vi "All Node Groups.vi"(8 "error in (no error)":errorcluster, 10 "Node Name":string, 11 "ChannelService in":refnum<class "ChannelService.lvclass">) -> (0 "error out":errorcluster, 2 "Node Groups":refnum<class "Group.lvclass">[](array[class]), 3 "ChannelService out":refnum<class "ChannelService.lvclass">)   [LabVIEW 2020, in "Vecto.lvlib" / "ChannelService.lvclass"]
uses:
  ChannelService.lvclass
  Group/Group.lvclass
  GroupsAbstractValue/GroupsAbstractValue.lvclass
  C:/dev/lv20CE/relink/lv-promises/Promises/Value/Value.lvclass
  Lookup Group Data.ctl
  Lookup Type.ctl
  lv-promises/Promises/Promise/Promise.lvclass
  ChannelService.lvclass/ChannelService.ctl
  lv-promises/Promises/Promise/Promise.lvclass/Promise.ctl
  lv-promises/Promises/Future/Future.lvclass/Future.ctl
  GroupsAbstractValue/GroupsAbstractValue.lvclass/GroupsAbstractValue.ctl
  lv-promises/Promises/Future/Future.lvclass
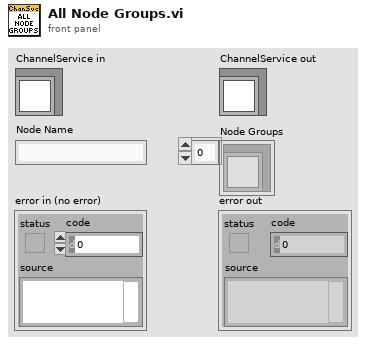
[diagram p1: front panel]
types:
  T1 = typedef "Vecto.lvlib/ChannelService.lvclass/Lookup Type.ctl" = enum16{"Name", "Node", "Pattern"}
  T2 = typedef "Vecto.lvlib/ChannelService.lvclass/Lookup Group Data.ctl" = cluster{"Type":T1, "Group Lookup":string, "Node Lookup":string, "Promise":refnum<class "Promise.lvclass">}
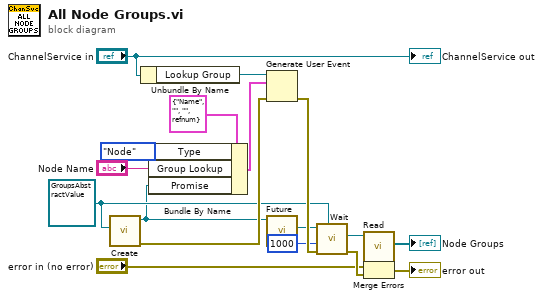
[diagram p0: block diagram]
diagram:
  w11 = refnum<class "GroupsAbstractValue.lvclass"> refnum ("Vecto.lvlib:GroupsValue.lvclass")
  n1 = call "Create.vi"("Result Type"=w11) -> ("error out"=w14:errorcluster, "Promise"=w6:refnum<class "Promise.lvclass">)  [unwired: 9 in]
  n2 = Unbundle By Name("ChannelService in") -> ("Lookup Group"=w13:refnum<user-event>)
  n3 = Bundle By Name(cluster=T2 {"Type"=enum."Name", "Group Lookup"="", "Node Lookup"="", "Promise"=refnum} ("Lookup Group Data"), "Type"=Lookup_Type."Node", "Group Lookup"="Node Name", "Promise"=w6) -> (w5:T2)
  n4 = Generate User Event(user event=w13, event data cluster=w5, error in=w14) -> (error out=w15:errorcluster)  [unwired: 1 in, 1 out]
  n5 = call "Future.vi"("Promise in"=w6) -> ("Future"=w12:refnum<class "Future.lvclass">)  [unwired: 9 in, 1 out]
  n6 = call "Wait.vi"("Result Type"=w11, "error in (no error)"=w15, "Timeout mS (-1)"=1000, "Future in"=w12) -> ("error out"=w17:errorcluster, "Result"=w9:refnum<class "GroupsAbstractValue.lvclass">)  [unwired: 6 in]
  n7 = call "Read.vi"("GroupsAbstractValue in"=w9) -> ("Groups"=→"Node Groups":refnum<class "Group.lvclass">[])  [unwired: 10 in]
  n8 = Merge Errors("error in (no error)", w17) -> (→"error out":errorcluster)
  "ChannelService out" <- "ChannelService in"
